vi "Get Last Bus Load.vi"(8 "error in (no error)":errorcluster, 11 "Load Calculator in":refnum<class "CANBus_Load_Calculator.lvclass">) -> (0 "error out":errorcluster, 2 "Bus Load (%)":dbl, 3 "Load Calculator out":refnum<class "CANBus_Load_Calculator.lvclass">)   [LabVIEW 2018, in "NI-XNET Monitor Engine.lvlib" / "XNET-Bus-Load-Calculator.lvlib"]
uses:
  XNET-Bus-Load-Calculator.lvlib
  CANBus/CANBus_Load_Calculator.lvclass
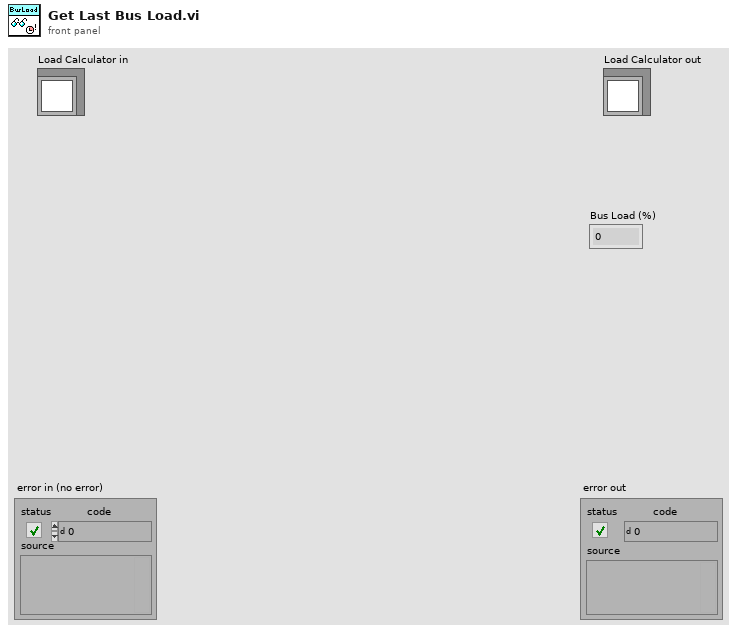
[diagram p1: front panel]
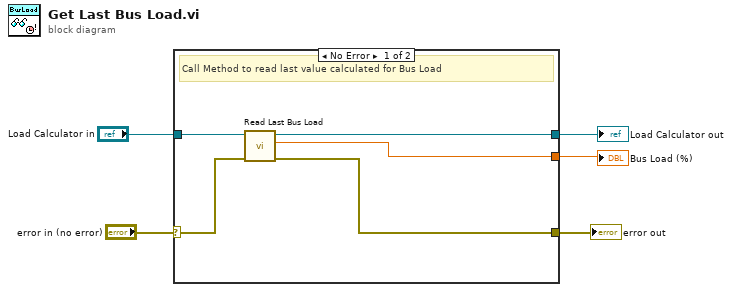
[diagram p0: block diagram]
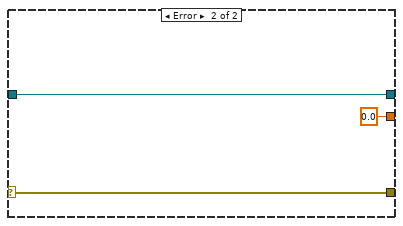
[diagram p2: hidden frame]
diagram:
  n1 = case shown="No Error" "error in (no error)" {
    selector: "error in (no error)" -> [w7 w13]
    tunnel: [w8 w13] -> w4
    tunnel: "Load Calculator in" -> [w10 w12]
    tunnel: [w9 w12] -> w2
    tunnel: [w6 0.0 ("Bus Load (%)")] -> w1
    frame No Error {
      # "Call Method to read last value calculated for Bus Load"
      n2 = call "Read Last Bus Load.vi"("error in (no error)"=w7, "GenBus_Load_Calculator in"=w10) -> ("error out"=w8:errorcluster, "Bus Load (%)"=w6:dbl, "GenBus_Load_Calculator out"=w9:refnum<class "CANBus_Load_Calculator.lvclass">)  [unwired: 7 in]
    }
    frame Error {
    }
  }
  "error out" <- w4
  "Load Calculator out" <- w2
  "Bus Load (%)" <- w1
